vi "Write HW Mods.vi"(8 "error in (no error)":errorcluster, 10 "HW Mods":string[](array[string]), 11 "Chassis BOM in":refnum<class "Chassis BOM.lvclass">) -> (0 "error out":errorcluster, 3 "Chassis BOM out":refnum<class "Chassis BOM.lvclass">)   [LabVIEW 2018, in "Configuration Grandmaster.lvlib" / "Chassis BOM.lvclass"]
uses:
  Chassis BOM.lvclass
  Chassis BOM.lvclass/Chassis BOM.ctl
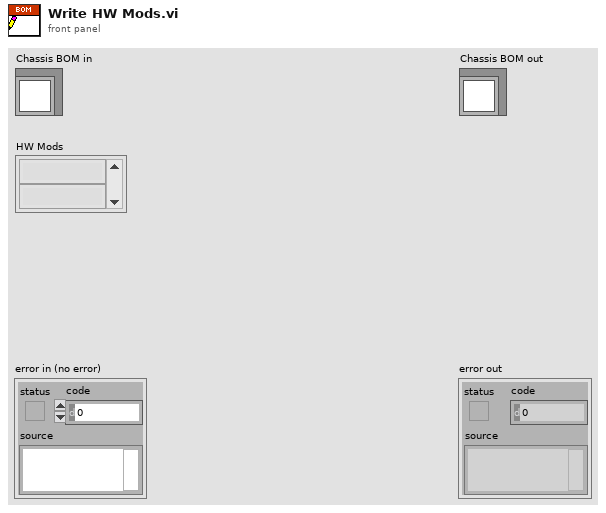
[diagram p1: front panel]
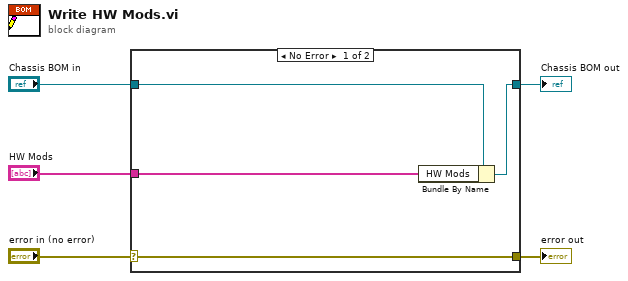
[diagram p0: block diagram]
diagram:
  n1 = case shown="No Error" "error in (no error)" {
    selector: "error in (no error)" -> [w9 w10]
    tunnel: [w9 w10] -> w4
    tunnel: [w7 w11] -> w2
    tunnel: "Chassis BOM in" -> [w8 w11]
    tunnel: "HW Mods" -> [w6 _]
    frame No Error {
      n2 = Bundle By Name(cluster=w8, "HW Mods"=w6) -> (w7:refnum<class "Chassis BOM.lvclass">)
    }
    frame Error {
    }
  }
  "error out" <- w4
  "Chassis BOM out" <- w2
